vi "FTW-Example-SLASD-Core-Initialize.vi"(0 "Initialization Sequence":string, 5 "FTW Actor Instance Configuration":string, 11 "error in (no error)":errorcluster) -> (4 "Actor Template-Core out":refnum<class "FTW-Example-SLASD-Core.lvclass">, 6 "Incoming Requests":refnum<event-registration>, 15 "error out":errorcluster)   [LabVIEW 2013, in "FTW-Example-SLASD-Core.lvclass"]
uses:
  FTW-Example-SLASD-Core.lvclass
  Actor/src/Message/Request/FTW-Message-IncomingRequest.lvclass
  Core/src/Reflection/FTW-Reflection-Type.vi
  Core/src/JSON/FTW-JSON-Core-LibraryFilepath.vi
  Core/src/JSON/FTW-JSON-Core-GetFlattenedValue.vi
  Core/src/JSON/FTW-JSON-Core-LibraryError.vi
  Core/utils/CodeGen/JSON Deserialize/FTW-JSON-Deserialize.xnode
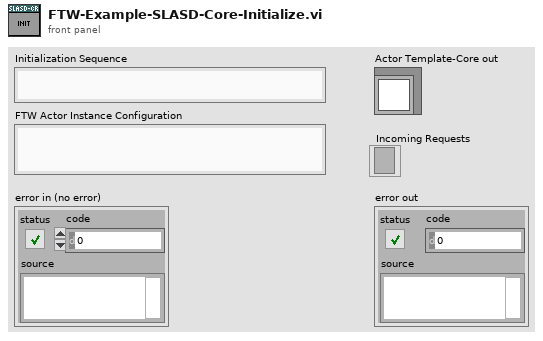
[diagram p1: front panel]
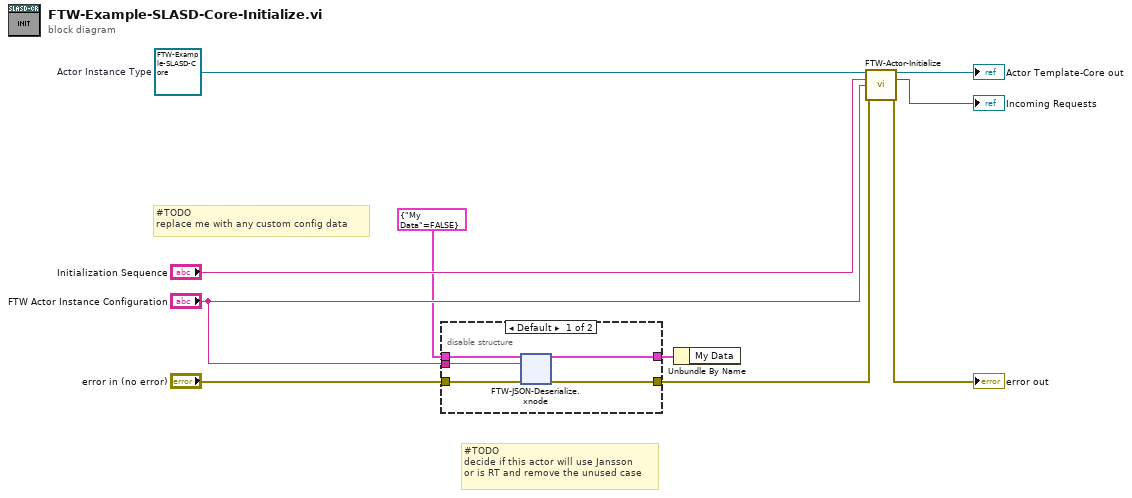
[diagram p0: block diagram]
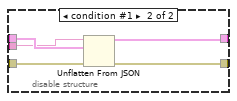
[diagram p2: hidden frame]
diagram:
  w1 = refnum<class "FTW-Example-SLASD-Core.lvclass"> refnum  # Actor Instance Type
  # "#TODO\ndecide if this actor will use Jansson\nor is RT and remove the unused case"
  # "#TODO\nreplace me with any custom config data"
  n1 = disable-structure shown="Default" {
    disable-tunnel: "error in (no error)" -> [w15 w54]
    disable-tunnel: [w14 w53] -> w5
    disable-tunnel: "FTW Actor Instance Configuration" -> [w13 w51]
    disable-tunnel: cluster{"My Data":bool} {"My Data"=FALSE} ("Type and Defaults") -> [w12 w52]
    disable-tunnel: [w11 w50] -> w2
    frame condition #0 (active) {
      n2 = xnode "FTW-JSON-Deserialize.xnode"("Type and Defaults"=w12, "JSON String"=w13, "error in"=w15) -> ("Values"=w11:cluster{"My Data":bool}, "error out"=w14:errorcluster)
    }
    frame condition #1 {
      n3 = Unflatten From JSON(JSON string=w51, type and defaults=w52, error in (no error)=w54) -> (value=w50:cluster{"My Data":bool}, error out=w53:errorcluster)  [unwired: 4 in]
    }
  }
  n4 = Unbundle By Name(w2) -> ()  [unwired: 1 out]
  n5 = call-dynamic "FTW-Actor-Initialize.vi"("FTW Actor Instance Type"=w1, "Initialization Job Sequence"="Initialization Sequence", "Actor Instance Configuration"="FTW Actor Instance Configuration", "error in"=w5) -> ("FTW Actor Instance"=→"Actor Template-Core out":refnum<class "FTW-Example-SLASD-Core.lvclass">, "Incoming Requests"=→"Incoming Requests":refnum<event-registration>, "error out"=→"error out":errorcluster)  [unwired: 9 in]
